vi "Tektronix_scope_ch.vi"(8 "channel":T1) -> ()   [LabVIEW 2020]
doc: "This example illustrates how to use autosetup and continuously acquires waveforms from a single channel using the following steps:\n\n1. Specify a valid VISA session. \n2. Specify a channel. \n3. Specify a time-out value for reading waveform.\n4. Run the VI. The graph displays the waveform you acquire."
uses:
  <extravilib>/ChannelInstances/Tag-bool/))Channel.ctl
  <extravilib>/ChannelInstances/Tag-bool/Read With Abort.vi
  <extravilib>/ChannelInstances/Tag-bool/EndpointRead.vi
  <instrlib>/Tektronix DPO MSO 2000 4000 Series/Public/Data/Read (Multiple Waveforms).vi
  <instrlib>/Tektronix DPO MSO 2000 4000 Series/Tektronix DPO MSO 2000 4000 Series.lvlib
  <extravilib>/ChannelInstances/Tag-bool.lvlib
panel:
  out "Waveform Graph":waveform(dbl)[](graph)
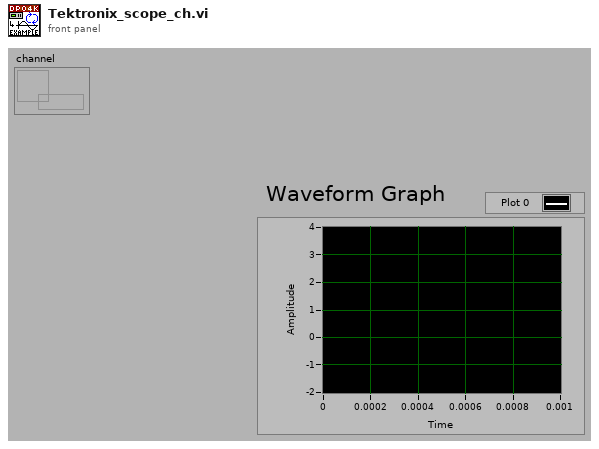
[diagram p1: front panel]
types:
  T1 = typedef "Tag-bool.lvlib/))Channel.ctl" = refnum<queue>
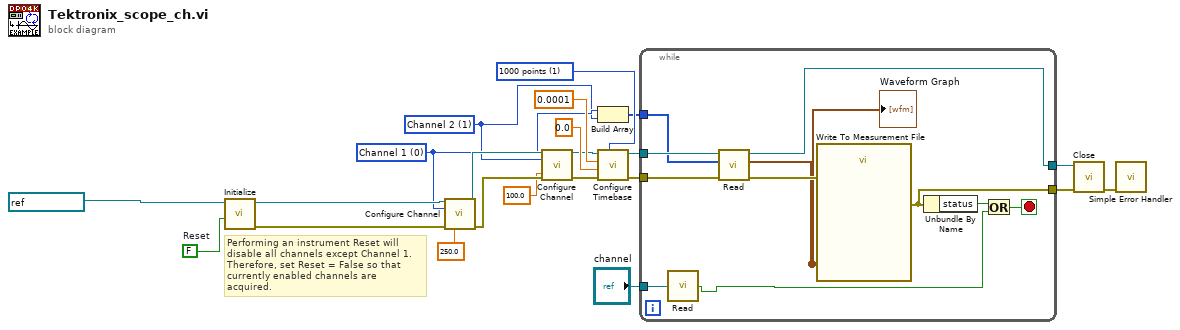
[diagram p0: block diagram]
diagram:
  w7 = u16 1 items=["Channel 1", "Channel 2", "Channel 3", "Channel 4", "Math", "Reference 1", "Reference 2", "Reference 3", "Reference 4", "Bus 1", "Bus 2"] ("Channel (0: Channel 1)")
  w8 = u16 0 items=["Channel 1", "Channel 2", "Channel 3", "Channel 4", "Math", "Reference 1", "Reference 2", "Reference 3", "Reference 4", "Bus 1", "Bus 2"] ("Channel (0: Channel 1)")
  w16 = u32 1 items=["1000 points"=1, "10k points"=10, "100k points"=100, "1M points"=1000, "5M points"=5000, "10M points"=10000] ("Record Length (10: 10k points)")
  w21 = FALSE  # Reset
  # "Performing an instrument Reset will disable all channels except Channel 1. Therefore, set Reset = False so that currently enabled channels are acquired."
  n1 = call <instrlib>:"Initialize.vi"("Reset (True)"=w21, "VISA resource name"=refnum<visa-resource-name> "MSO3014") -> ("error out"=w12:errorcluster, "VISA resource name out"=w13:refnum<visa-resource-name>)  [unwired: 8 in]
  n2 = call <instrlib>:"Configure Channel.vi"("VISA resource name"=w13, "Channel (0: Channel 1)"=w8, "error in (no error)"=w12, "Vertical Range (10.0 V)"=250.0) -> ("VISA resource name out"=w11:refnum<visa-resource-name>, "error out"=w10:errorcluster)  [unwired: 10 in]
  n3 = call <instrlib>:"Configure Channel.vi"("VISA resource name"=w11, "Channel (0: Channel 1)"=w7, "error in (no error)"=w10, "Vertical Range (10.0 V)"=100.0) -> ("VISA resource name out"=w6:refnum<visa-resource-name>, "error out"=w5:errorcluster)  [unwired: 10 in]
  n4 = Build Array(w8, w7) -> (w9:u16[])
  n5 = call <instrlib>:"Configure Timebase.vi"("Record Length (10: 10k points)"=w16, "error in (no error)"=w5, "Position (10 %)"=0.0, "Timebase (0.0005 s)"=0.0001, "VISA resource name"=w6) -> ("error out"=w19:errorcluster, "VISA resource name out"=w20:refnum<visa-resource-name>)  [unwired: 5 in]
  n6 = while {
    tunnel: w20 -> [w33]
    tunnel: w19 -> [w32]
    tunnel: [w29] -> w15
    tunnel: [w31] -> w14
    tunnel: w9 -> [w27]
    tunnel: "channel" -> [w23]
    stop <- w25 stop-if-true
    n7 = call <instrlib>:"Read.vi"("channel"=w23) -> ("element"=w24:bool)  [unwired: 1 in, 1 out]
    n8 = call-poly <instrlib>:"Read.vi"("error in (no error)"=w32, "Channels"=w27, "VISA resource name"=w33) -> ("error out"=w28:errorcluster, "Waveform Data"=w26:waveform(dbl)[], "VISA resource name out"=w31:refnum<visa-resource-name>)  [unwired: 6 in]
    "Waveform Graph" <- w26
    n9 = call "Write To Measurement File"("Signals"=w26, "error in (no error)"=w28) -> ("error out"=w29:errorcluster)  [unwired: 15 in, 2 out]
    n10 = Unbundle By Name(w29) -> ("status"=w30:bool)
    n11 = Or(x=w30, y=w24) -> (x .or. y?=w25:bool)
  }
  n12 = call <instrlib>:"Close.vi"("error in (no error)"=w15, "VISA resource name"=w14) -> ("error out"=w22:errorcluster)  [unwired: 9 in]
  n13 = call <vilib>:"Simple Error Handler.vi"("error in (no error)"=w22) -> ()  [unwired: 4 in, 5 out]
